vi "LED STATUS.vi"(8 "error in (no error)":errorcluster, 11 "LOOP (ms)":u32=50) -> (0 "error out":errorcluster)   [LabVIEW 2023]
uses:
  ctrl defs/ctrl LED STATES.ctl
  <vilib>/Rock Robotics/WPI/DriverStation/WPI_DriverStationRobotMode2.ctl
  <vilib>/Rock Robotics/WPI/DriverStation/WPI_DriverStationAllianceInfo.ctl
  ctrl defs/ctrl LED PATTERN DEFS.ctl
  Global INIT.vi
  Global stack names.vi
  <vilib>/Rock Robotics/Network Tables/NT Read Boolean.vi
  Global odometry.vi
panel:
  in  "AUTO DEFAULT":T1=enum."COLOR 1 scan COLOR 2"
  in  "EMERGENCY STOP":T1=enum."COLOR 1 scan COLOR 2"
  in  "ARMS LOCKED":T1=enum."CROSSING, RED & BLUE"
  in  "PUKE":T1=enum."PINK, SOLID"
  in  "LOOKING for NOTE":T1=enum."RED, SCAN"
  in  "NOTE LOADED":T1=enum."GREEN, BLINK"
  in  "END GAME 2":T1=enum."RED, EX-CON"
  in  "END GAME 1":T1=enum."BLUE, EX-CON"
  in  "LOW BATT":T1=enum."RED, SOLID"
  in  "SELECT  AMP":T1=enum."ORANGE, BUMPER"
  in  "FIRE":T1=enum."ORANGE, BLINK"
  in  "DEFAULT":T1=enum."COLOR 1 scan COLOR 2"
  out "Teleop indicators":T2
  in  "pattern":T1=enum."COLOR 1 scan COLOR 2"
  in  "manual\noveride":bool
  out "Alliance":T3
  out "Robot Mode":T4=enum."Teleop Enabled"
  out "Match Time(s)":sgl=-1.0
  out "LED state":T5=enum."WRITE LED VALUE"
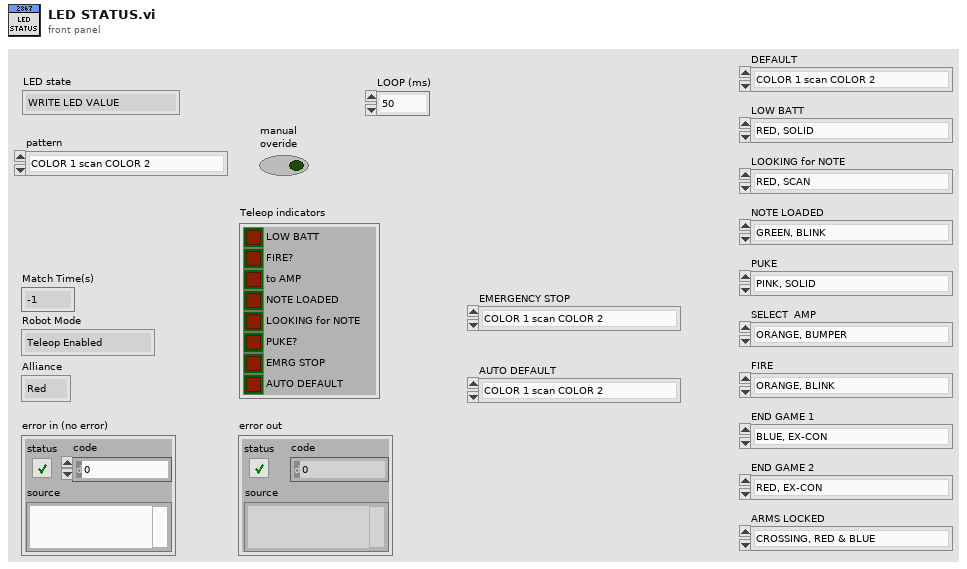
[diagram p1: front panel]
types:
  T1 = typedef "ctrl LED PATTERN DEFS.ctl" = enum16{"default", "RED, SOLID", "RED, BUMPER", "RED, BLINK", "RED, WAVE", "RED, SCAN", "RED, PULSE", "BLUE, SOLID", "BLUE, BUMPER", "BLUE, BLINK", "BLUE, WAVE", "BLUE, SCAN", "BLUE, PULSE", "GREEN, SOLID", "GREEN, BUMPER", "GREEN, BLINK", "GREEN, WAVE", "GREEN, SCAN", "GREEN, PULSE", "WHITE, WAVE", "WHITE, PULSE", "COLOR 1 scan white", "COLOR 1 scan COLOR 2", "COLOR 1 bumper white", "COLOR 1 bumper COLOR 2", "PINK, SOLID", "PINK, BLINK", "VIOLET, SOLID", "VIOLET, BLINK", "ORANGE, SOLID", "ORANGE, BLINK", "YELLOW, SOLID", "YELLOW, BLINK", "FUSCIA, SOLID", "FUSCIA, BLINK", "AQUA, SOLID", "AQUA, BLINK", "AQUA, BUMPER", "AQUA, SCAN", "FUSCIA, BUMPER", "FUSCIA, SCAN", "ORANGE, BUMPER", "ORANGE, SCAN", "VIOLET, BUMPER", "VIOLET, SCAN", "YELLOW, BUMPER", "YELLOW, SCAN", "PINK, BUMPER", "PINK, SCAN", "CROSSING, RED & BLUE", "CROSSING, COLORS 1&2", "TEST", "RAINBOW", "RED, EXPAND", "BLUE, EXPAND", "GREEN, EXPAND", "RED, EX-CON", "BLUE, EX-CON", "GREEN, EX-CON", "EMERGENCY STOP", "LOW BATTERY"}
  T2 = cluster{"LOW BATT":bool, "FIRE?":bool, "to AMP":bool, "NOTE LOADED":bool, "LOOKING for NOTE":bool, "PUKE?":bool, "EMRG STOP":bool, "AUTO DEFAULT":bool}
  T3 = typedef "WPI_DriverStationAllianceInfo.ctl" = enum16{"Red", "Blue", "Invalid"}
  T4 = typedef "WPI_DriverStationRobotMode2.ctl" = enum16{"Autonomous Disabled", "Autonomous Enabled", "Teleop Disabled", "Teleop Enabled", "Disconnected", "Finish", "Test Disabled", "Test Enabled", "Emergency Stopped"}
  T5 = typedef "ctrl LED STATES.ctl" = enum16{"STANDBY", "END GAME 1", "END GAME 2", "NOTE is LOADED", "LOOKING for NOTE", "PUKE", "FIRE", "SHOOT AMP", "EXTENDING ARMS", "RETRACTING ARMS", "ARMS LOCKED", "LOW BATTERY", "WRITE LED VALUE", "DEFAULT PATTERN", "EMERGENCY STOP", "AUTO DEFAULT"}
  T6 = typedef "ctrl LED init.ctl" = cluster{"PWM Channel":T7, "refnum name":string, "#LEDS":T8, "initial output":dbl, "stack name":string, "Installed?":bool, "pattern":T9}
  T7 = typedef "FPGA_DIOPWMChannel.ctl" = enum8{"PWM 0", "PWM 1", "PWM 2", "PWM 3", "PWM 4", "PWM 5", "PWM 6", "PWM 7", "PWM 8", "PWM 9", "PWM MXP 0", "PWM MXP 1", "PWM MXP 2", "PWM MXP 3", "PWM MXP 4", "PWM MXP 5", "PWM MXP 6", "PWM MXP 7", "PWM MXP 8", "PWM MXP 9", "Invalid"}
  T8 = typedef "ctrl number of LEDs.ctl" = u16
  T9 = typedef "ctrl LED PATTERNS.ctl" = u16
  T10 = typedef "ctrl stack - INTAKE SHOOTER.ctl" = cluster{"INTAKE STATE":string, "RUN INTAKE?":string, "RUN REVERSE?":string, "NOTE LOADED?":string, "SHOOTER STATE":string, "SHOOTER FIRE?":string, "SHOOT AMP?":string, "EXTEND FLAP?":string, "LOOKING for NOTE":string, "OVERIDE NOTE CHECK":string}
  T11 = cluster{"Battery Voltage Fault":bool, "Hardware Fault":bool, "CAN Warning Fault":bool, "Temperature Fault":bool}
  T12 = cluster{"Brownout":bool, "CAN Warning":bool, "Can Bus Off":bool, "Hardware Fault":bool, "Firmware Fault":bool, "CH20 Brownout":bool, "CH21 Brownout":bool, "CH22 Brownout":bool, "CH23 Brownout":bool, "Has Reset":bool}
  T13 = cluster{"LEFT ARM":cluster{"VBus%":dbl, "LOCK?":bool, "LOCKED":bool}, "RIGHT ARM":cluster{"VBus%":dbl, "LOCK?":bool, "LOCKED":bool}}
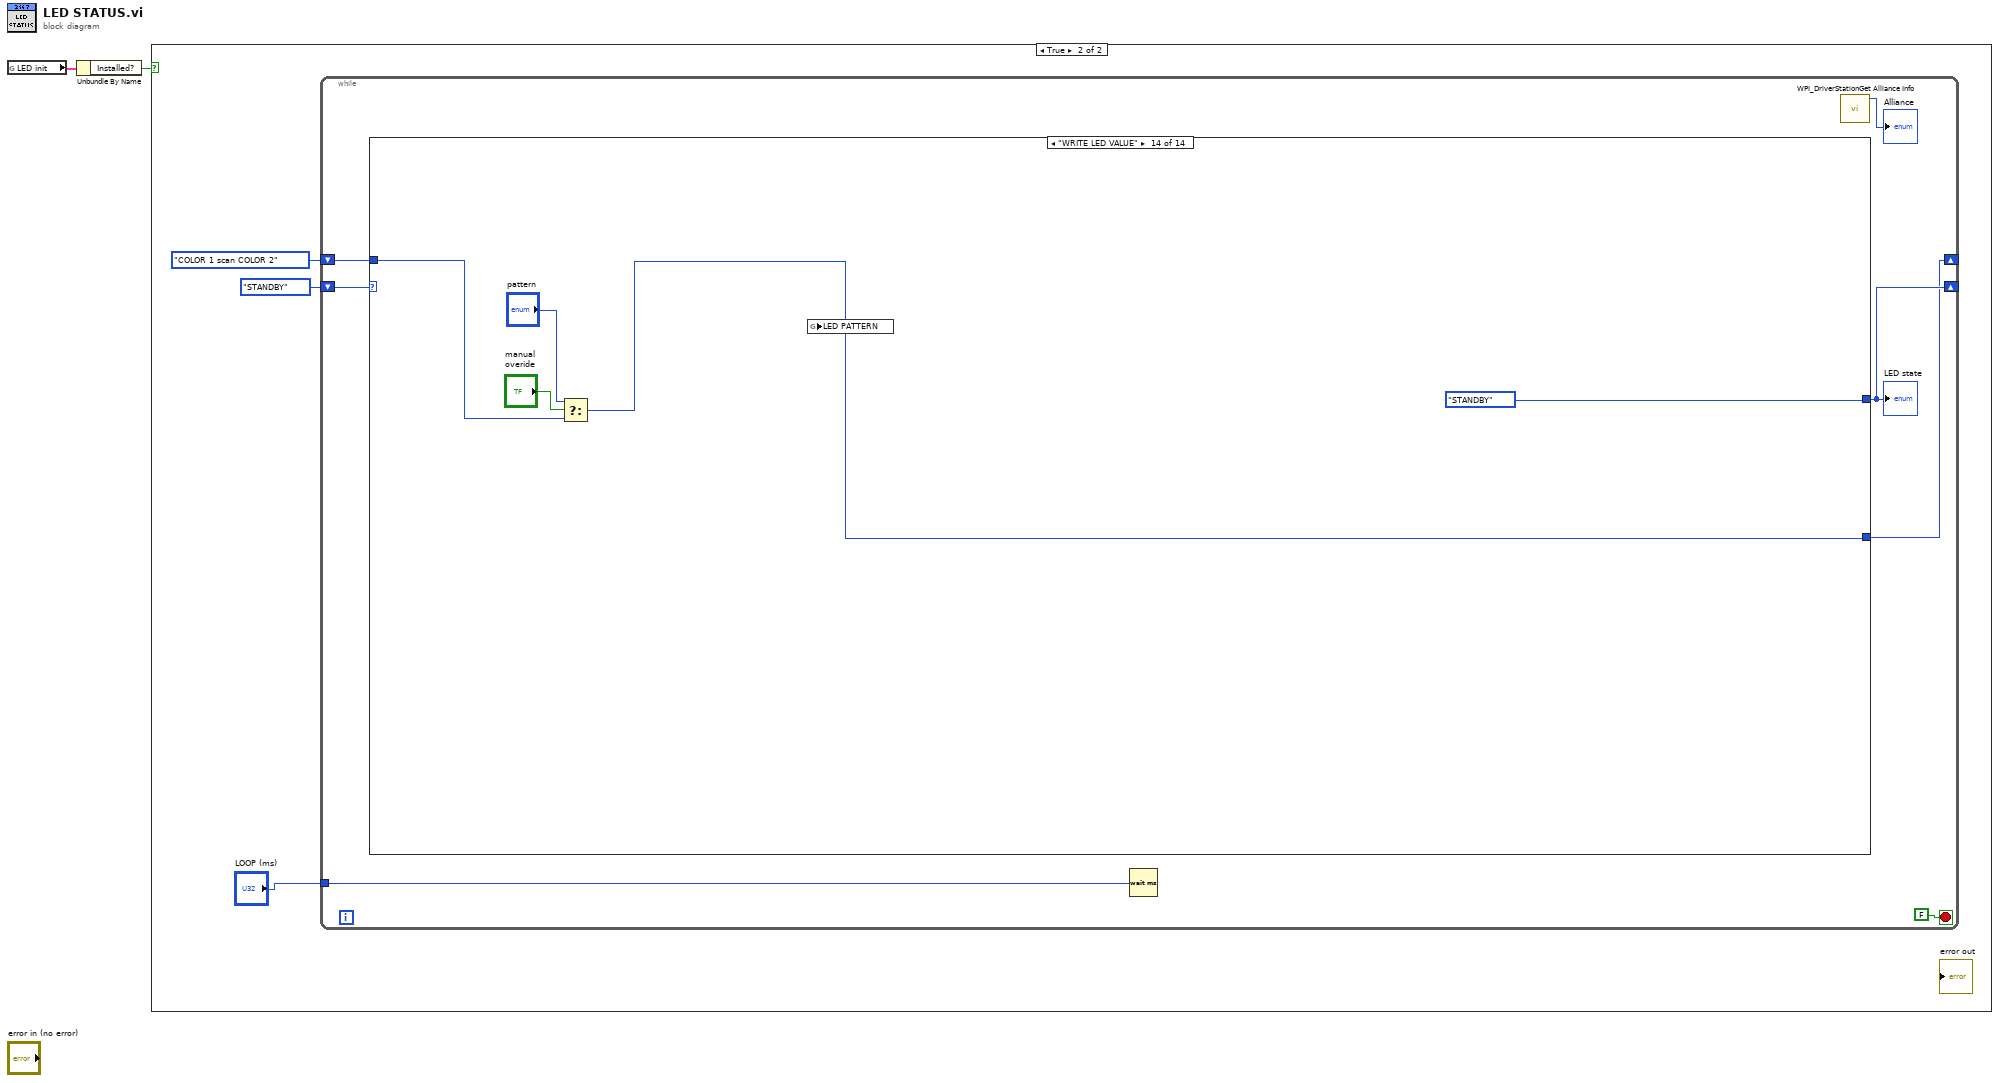
[diagram p0: block diagram]
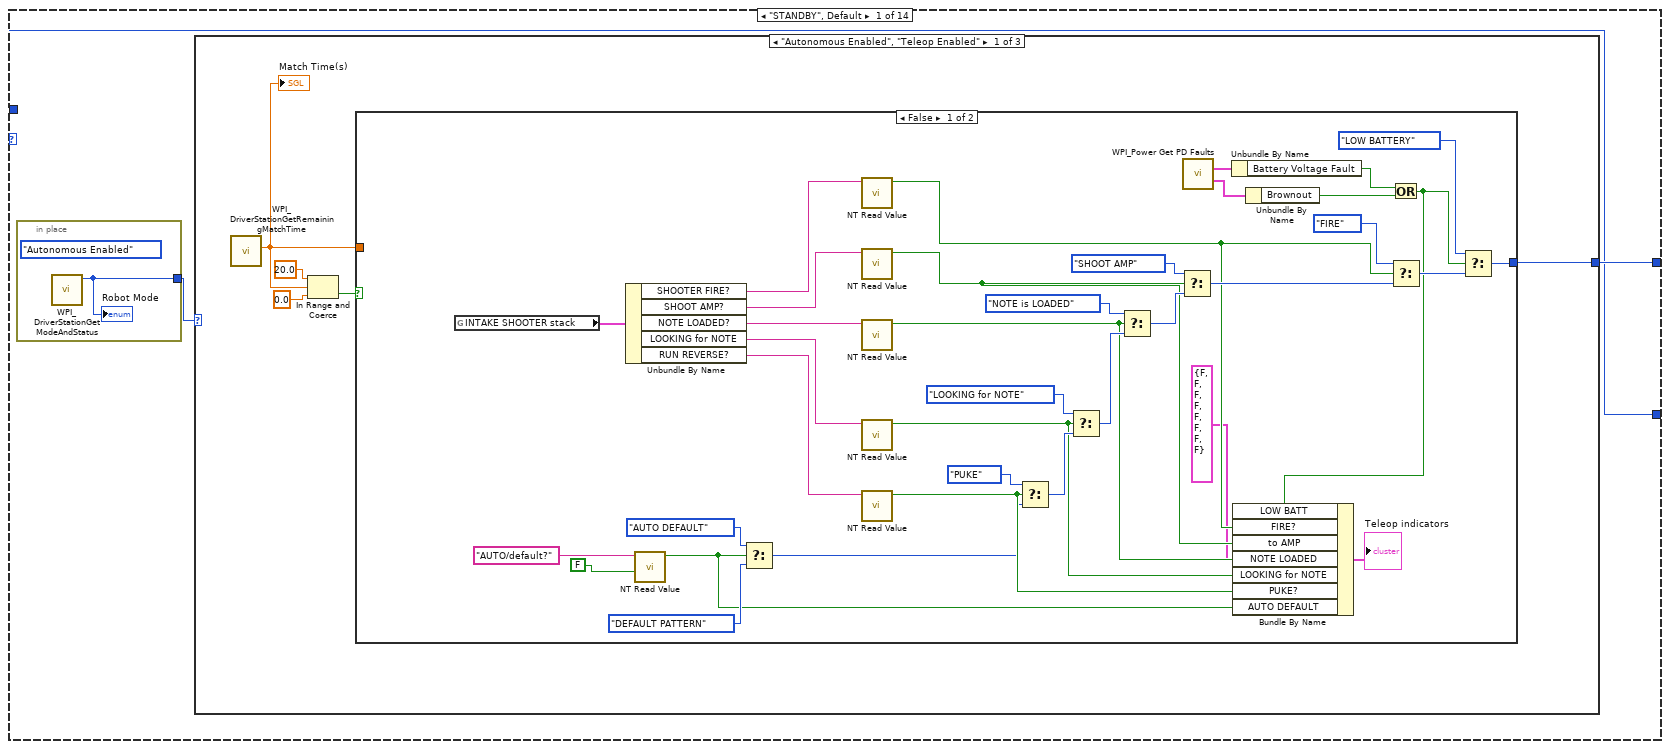
[diagram p3: hidden frame]
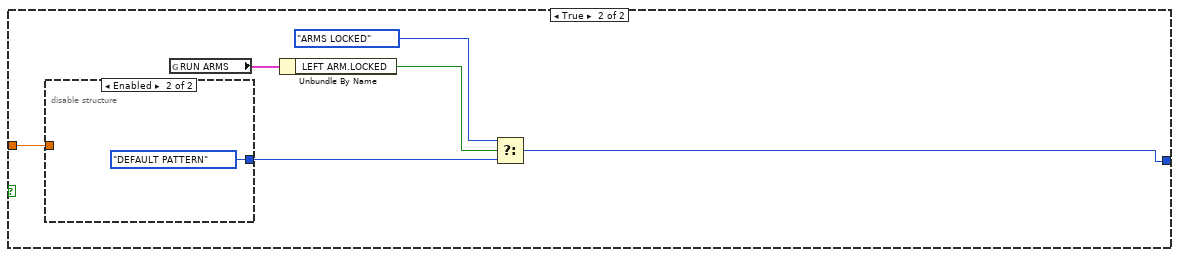
[diagram p4: hidden frame]
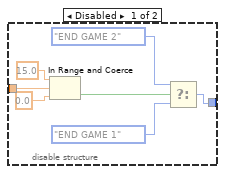
[diagram p5: hidden frame]
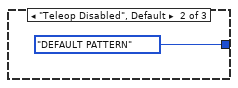
[diagram p6: hidden frame]
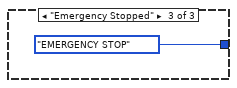
[diagram p7: hidden frame]
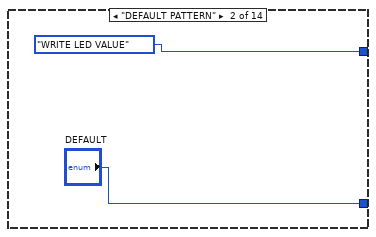
[diagram p8: hidden frame]
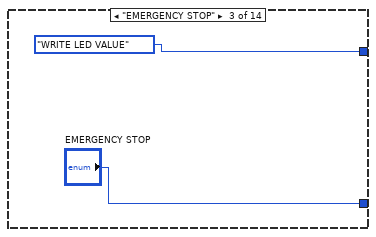
[diagram p9: hidden frame]
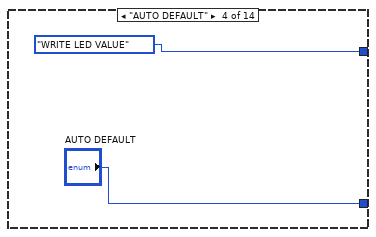
[diagram p10: hidden frame]
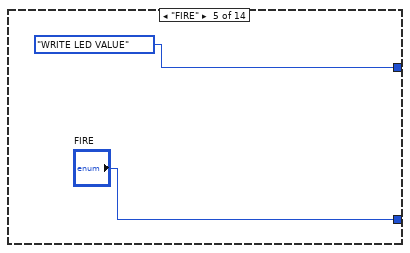
[diagram p11: hidden frame]
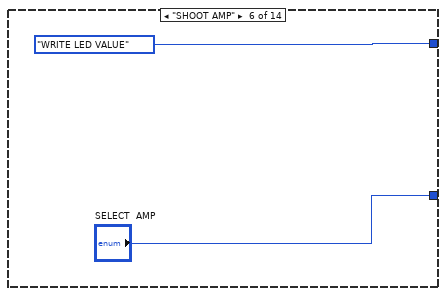
[diagram p12: hidden frame]
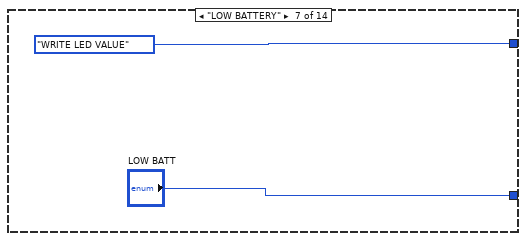
[diagram p13: hidden frame]
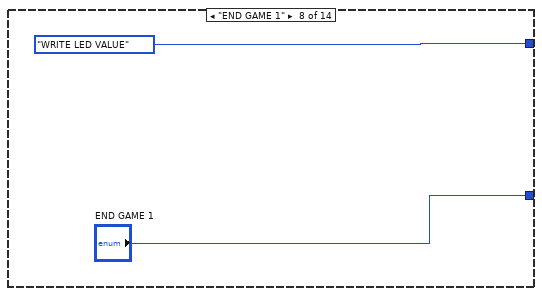
[diagram p14: hidden frame]
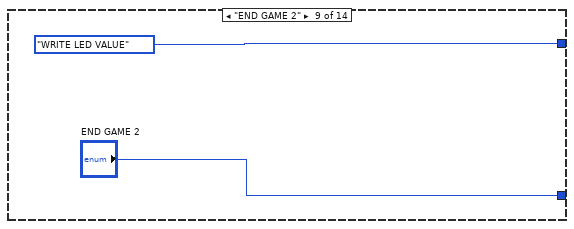
[diagram p15: hidden frame]
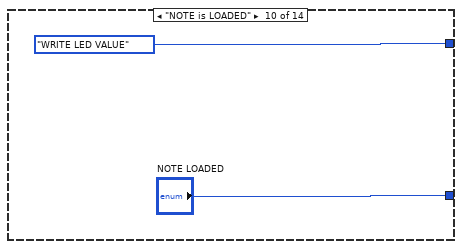
[diagram p16: hidden frame]
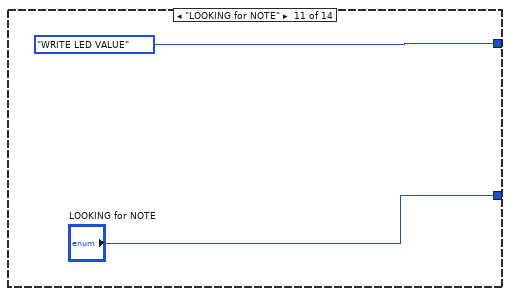
[diagram p17: hidden frame]
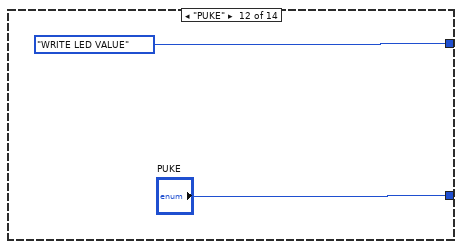
[diagram p18: hidden frame]
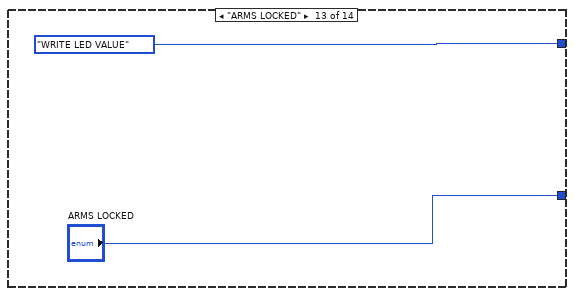
[diagram p19: hidden frame]
diagram:
  n1 = global read "Global INIT.vi" "LED init"() -> (w1:T6)
  n2 = Unbundle By Name(w1) -> ("Installed?"=w2:bool)
  n3 = case shown="True" w2 {
    frame False {
    }
    frame True {
      n4 = while {
        shift-right: [w11] -> _
        shift-left: ctrl_LED_STATES."STANDBY" -> [w8]
        shift-right: [w7] -> _
        shift-left: ctrl_LED_PATTERN_DEFS."COLOR 1 scan COLOR 2" ("pattern") -> [w10]
        tunnel: "LOOP (ms)" -> [w6]
        stop <- FALSE stop-if-true
        n5 = case shown="\"WRITE LED VALUE\"" w8 {
          tunnel: [w15 ctrl_LED_STATES."WRITE LED VALUE" ctrl_LED_STATES."WRITE LED VALUE" ctrl_LED_STATES."WRITE LED VALUE" ctrl_LED_STATES."WRITE LED VALUE" ctrl_LED_STATES."WRITE LED VALUE" ctrl_LED_STATES."WRITE LED VALUE" ctrl_LED_STATES."WRITE LED VALUE" ctrl_LED_STATES."WRITE LED VALUE" ctrl_LED_STATES."WRITE LED VALUE" ctrl_LED_STATES."WRITE LED VALUE" ctrl_LED_STATES."WRITE LED VALUE" ctrl_LED_STATES."WRITE LED VALUE" ctrl_LED_STATES."STANDBY"] -> w11
          tunnel: [w14 "DEFAULT" "EMERGENCY STOP" "AUTO DEFAULT" "FIRE" "SELECT  AMP" "LOW BATT" "END GAME 1" "END GAME 2" "NOTE LOADED" "LOOKING for NOTE" "PUKE" "ARMS LOCKED" w98] -> w7
          tunnel: w10 -> [w14 _ _ _ _ _ _ _ _ _ _ _ _ w99]
          frame "STANDBY", Default {
            n6 = in-place {
              in-place-border: [w16] -> w13
              (unwired) WPI_DriverStationRobotMode2."Autonomous Enabled" ("Robot Mode")
              n7 = call <vilib>:"WPI_DriverStationGetModeAndStatus.vi"() -> ("Robot Mode"=w16:T4)  [unwired: 10 in, 1 out]
              "Robot Mode" <- w16
            }
            n8 = case shown="\"Autonomous Enabled\", \"Teleop Enabled\"" w13 {
              tunnel: [w21 ctrl_LED_STATES."DEFAULT PATTERN" ctrl_LED_STATES."EMERGENCY STOP"] -> w15
              frame "Autonomous Enabled", "Teleop Enabled" {
                n9 = call <vilib>:"WPI_DriverStationGetRemainingMatchTime.vi"() -> ("Match Time(s)"=w18:sgl)  [unwired: 10 in, 1 out]
                "Match Time(s)" <- w18
                n10 = In Range and Coerce(upper limit=20.0, x=w18, lower limit=0.0) -> (In Range?=w17:bool)  [unwired: 1 out]
                n11 = case shown="False" w17 {
                  tunnel: [w40 w61] -> w21
                  tunnel: w18 -> [_ w59]
                  frame False {
                    n12 = global read "Global stack names.vi" "INTAKE SHOOTER stack"() -> (w57:T10)
                    n13 = Unbundle By Name(w57) -> ("SHOOTER FIRE?"=w56:string, "SHOOT AMP?"=w55:string, "NOTE LOADED?"=w54:string, "LOOKING for NOTE"=w53:string, "RUN REVERSE?"=w52:string)
                    n14 = call-poly <vilib>:"NT Read Value.vi"("default value"=FALSE ("value"), "name"="AUTO/default?") -> ("value"=w22:bool)  [unwired: 7 in, 2 out]
                    n15 = Select(t=ctrl_LED_STATES."AUTO DEFAULT", s=w22, f=ctrl_LED_STATES."DEFAULT PATTERN") -> (s? t:f=w27:T5)
                    n16 = call-poly <vilib>:"NT Read Value.vi"("name"=w56) -> ("value"=w34:bool)  [unwired: 8 in, 2 out]
                    n17 = call-poly <vilib>:"NT Read Value.vi"("name"=w55) -> ("value"=w33:bool)  [unwired: 8 in, 2 out]
                    n18 = call-poly <vilib>:"NT Read Value.vi"("name"=w54) -> ("value"=w32:bool)  [unwired: 8 in, 2 out]
                    n19 = call-poly <vilib>:"NT Read Value.vi"("name"=w53) -> ("value"=w31:bool)  [unwired: 8 in, 2 out]
                    n20 = call-poly <vilib>:"NT Read Value.vi"("name"=w52) -> ("value"=w30:bool)  [unwired: 8 in, 2 out]
                    n21 = Select(t=ctrl_LED_STATES."PUKE", s=w30, f=w27) -> (s? t:f=w45:T5)
                    n22 = Select(t=ctrl_LED_STATES."LOOKING for NOTE", s=w31, f=w45) -> (s? t:f=w46:T5)
                    n23 = Select(t=ctrl_LED_STATES."NOTE is LOADED", s=w32, f=w46) -> (s? t:f=w48:T5)
                    n24 = Select(t=ctrl_LED_STATES."SHOOT AMP", s=w33, f=w48) -> (s? t:f=w50:T5)
                    n25 = call <vilib>:"WPI_Power Get PD Faults.vi"() -> ("Faults"=w42:T11, "Sticky Faults"=w41:T12)  [unwired: 12 in, 2 out]
                    n26 = Unbundle By Name(w42) -> ("Battery Voltage Fault"=w38:bool)
                    n27 = Unbundle By Name(w41) -> ("Brownout"=w37:bool)
                    n28 = Or(x=w38, y=w37) -> (x .or. y?=w35:bool)
                    n29 = Bundle By Name(cluster=T2 {"LOW BATT"=FALSE, "FIRE?"=FALSE, "to AMP"=FALSE, "NOTE LOADED"=FALSE, "LOOKING for NOTE"=FALSE, "PUKE?"=FALSE, "EMRG STOP"=FALSE, "AUTO DEFAULT"=FALSE} ("Teleop indicators"), "LOW BATT"=w35, "FIRE?"=w34, "to AMP"=w33, "NOTE LOADED"=w32, "LOOKING for NOTE"=w31, "PUKE?"=w30, "AUTO DEFAULT"=w22) -> (→"Teleop indicators":T2)
                    n30 = Select(t=ctrl_LED_STATES."FIRE", s=w34, f=w50) -> (s? t:f=w39:T5)
                    n31 = Select(t=ctrl_LED_STATES."LOW BATTERY", s=w35, f=w39) -> (s? t:f=w40:T5)
                  }
                  frame True {
                    n32 = disable-structure shown="Enabled" {
                      disable-tunnel: w59 -> [w65 _]
                      disable-tunnel: [w64 ctrl_LED_STATES."DEFAULT PATTERN"] -> w58
                      frame Disabled {
                        n33 = In Range and Coerce(upper limit=sgl 15.0 ("y"), x=w65, lower limit=sgl 0.0) -> (In Range?=w70:bool)  [unwired: 1 out]
                        n34 = Select(t=ctrl_LED_STATES."END GAME 2", s=w70, f=ctrl_LED_STATES."END GAME 1") -> (s? t:f=w64:T5)
                      }
                      frame Enabled {
                      }
                    }
                    n35 = global read "Global odometry.vi" "RUN ARMS"() -> (w60:T13)
                    n36 = Unbundle By Name(w60) -> ("LEFT ARM.LOCKED"=w63:bool)
                    n37 = Select(t=ctrl_LED_STATES."ARMS LOCKED", s=w63, f=w58) -> (s? t:f=w61:T5)
                  }
                }
              }
              frame "Teleop Disabled", Default {
              }
              frame "Emergency Stopped" {
              }
            }
          }
          frame "DEFAULT PATTERN" {
          }
          frame "EMERGENCY STOP" {
          }
          frame "AUTO DEFAULT" {
          }
          frame "FIRE" {
          }
          frame "SHOOT AMP" {
          }
          frame "LOW BATTERY" {
          }
          frame "END GAME 1" {
          }
          frame "END GAME 2" {
          }
          frame "NOTE is LOADED" {
          }
          frame "LOOKING for NOTE" {
          }
          frame "PUKE" {
          }
          frame "ARMS LOCKED" {
          }
          frame "WRITE LED VALUE" {
            n38 = Select(t="pattern", s="manual\noveride", f=w99) -> (s? t:f=w98:T1)
            n39 = global write "Global odometry.vi" "LED PATTERN"(w98) -> ()
          }
        }
        "LED state" <- w11
        n40 = Wait (ms)(milliseconds to wait=w6) -> ()  [unwired: 1 out]
        n41 = call <vilib>:"WPI_DriverStationGet Alliance Info.vi"() -> ("Alliance"=→"Alliance":T3)  [unwired: 6 in, 5 out]
      }
    }
  }
